vi "New.vi"() -> ()   [LabVIEW 2020, in "MeasurementService Editor.lvlib"]
uses:
  _Editor/MeasurementService Editor.lvlib
panel:
  out "Status":string
  in  "Create Measurement Service":bool
  in  "Measurement Service Name":string
  out "Active Project Name":string
  # "* Project in which Measurement Service will be created"
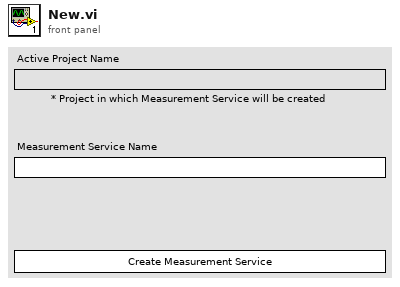
[diagram p1: front panel]
types:
  T1 = enum8{"Enabled", "Disabled", "Disabled and Grayed Out"}
  T2 = cluster{"Project ref":refnum<vi>, "Measurement Service Name":string}
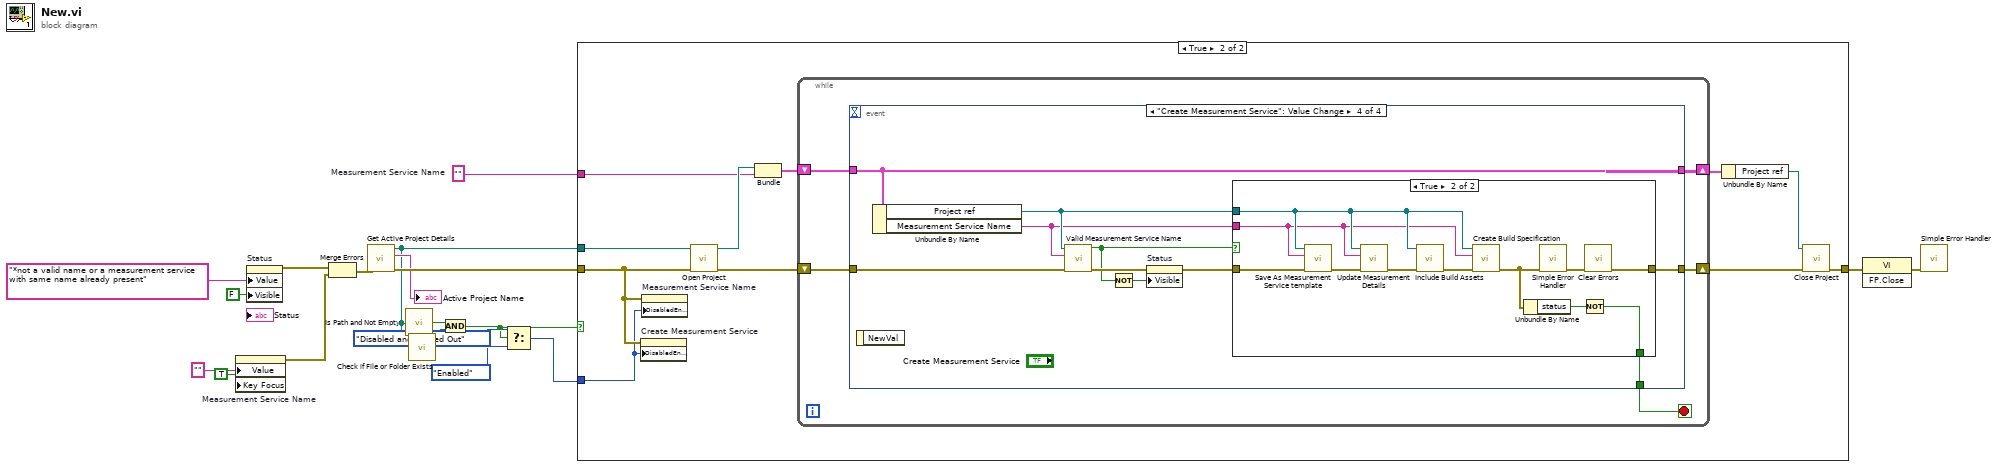
[diagram p0: block diagram]
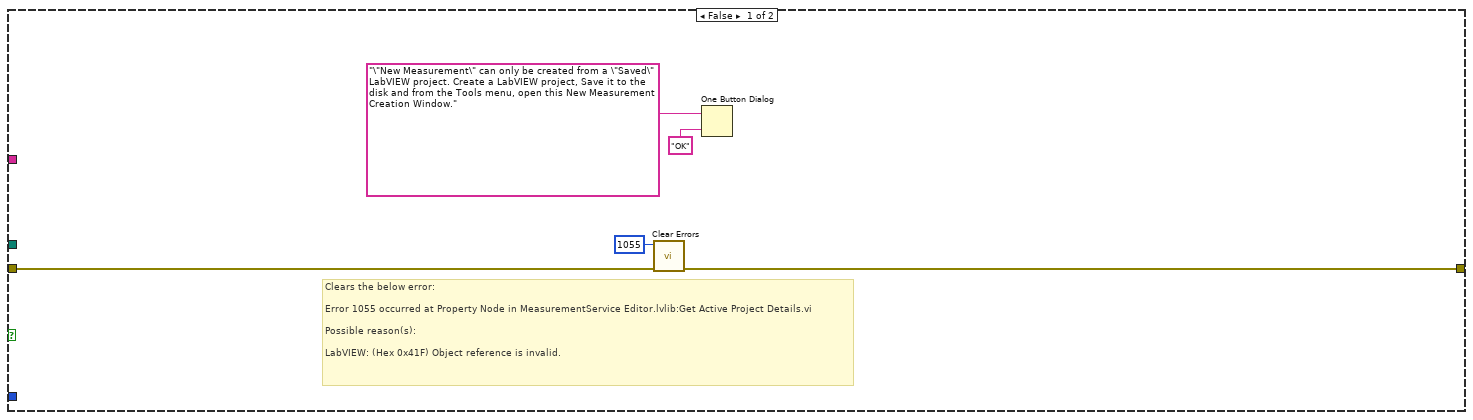
[diagram p2: hidden frame]
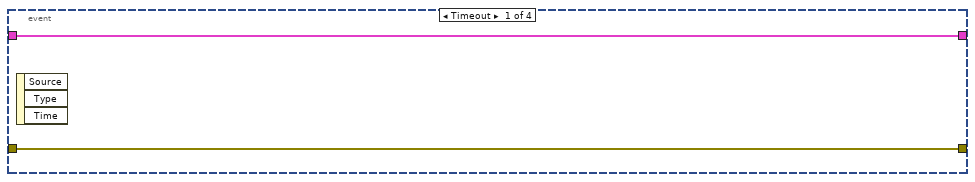
[diagram p3: hidden frame]
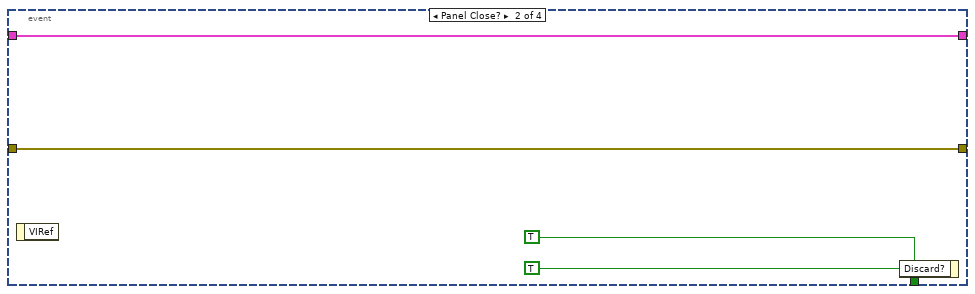
[diagram p4: hidden frame]
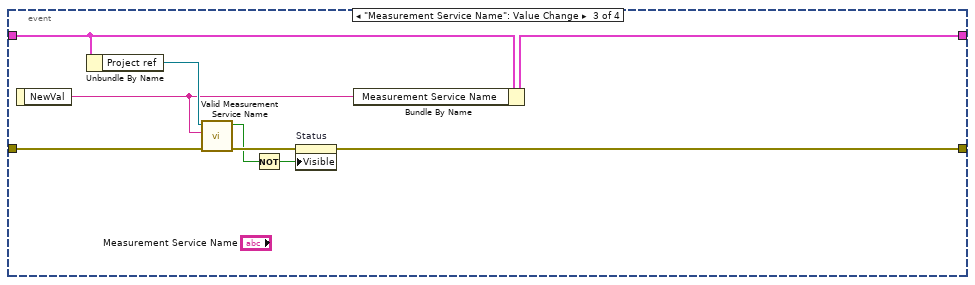
[diagram p5: hidden frame]
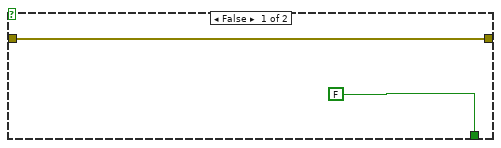
[diagram p6: hidden frame]
diagram:
  w19 = ""  # Measurement Service Name
  n1 = property on="Measurement Service Name" class="Str"("Value"="" ("Measurement Service Name"), "Key Focus"=TRUE) -> (error out=w14:errorcluster)  [unwired: 2 in, 1 out]
  n2 = property on="Status" class="Str"("Value"="*not a valid name or a measurement service with same name already present" ("Status"), "Visible"=FALSE) -> (error out=w16:errorcluster)  [unwired: 2 in, 1 out]
  n3 = Merge Errors(w16, w14) -> (w15:errorcluster)
  n4 = call "Get Active Project Details.vi"("error in"=w15) -> ("error out"=w10:errorcluster, "Name"=→"Active Project Name":string, "Path"=w5:path)  [unwired: 8 in]
  n5 = call <vilib>:"Is Path and Not Empty.vi"("path"=w5) -> ("Is Path and Not Empty?"=w4:bool)  [unwired: 4 in]
  n6 = call <vilib>:"Check if File or Folder Exists.vi"("path"=w5) -> ("file or folder exists?"=w3:bool)  [unwired: 8 in, 2 out]
  n7 = And(x=w4, y=w3) -> (x .and. y?=w2:bool)
  n8 = Select(t=T1."Enabled" ("Disabled"), s=w2, f=T1."Disabled and Grayed Out" ("Disabled")) -> (s? t:f=w6:T1)
  n9 = case shown="True" w2 {
    tunnel: w19 -> [_ w29]
    tunnel: [w21 w28] -> w12
    tunnel: w10 -> [w24 w27]
    tunnel: w6 -> [_ w26]
    tunnel: w5 -> [_ w25]
    frame False {
      # "Clears the below error:\n\nError 1055 occurred at Property Node in MeasurementService Editor.lvlib:Get Active Project Details.vi\n\nPossible reason(s):\n\nLabVIEW: (Hex 0x41F) Object reference is invalid."
      n10 = call <vilib>:"Clear Errors.vi"("error in (no error)"=w24, "specific error code to clear (0: all)"=1055) -> ("error out"=w21:errorcluster)  [unwired: 4 in, 1 out]
      n11 = One Button Dialog(message="\"New Measurement\" can only be created from a \"Saved\" LabVIEW project. Create a LabVIEW project, Save it to the disk and from the Tools menu, open this New Measurement Creation Window.", button name ("OK")="OK") -> ()  [unwired: 1 out]
    }
    frame True {
      n12 = property on="Create Measurement Service" class="Bool"(error in=w27, "DisabledEnum"=w26) -> ()  [unwired: 1 in, 2 out]
      n13 = property on="Measurement Service Name" class="Str"(error in=w27, "DisabledEnum"=w26) -> ()  [unwired: 1 in, 2 out]
      n14 = call "Open Project.vi"("error in"=w27, "Path"=w25) -> ("error out"=w35:errorcluster, "Project ref"=w34:refnum<vi>)  [unwired: 8 in]
      n15 = Bundle("Project ref"=w34, "Measurement Service Name"=w29) -> (w33:T2)  [unwired: 1 in]
      n16 = while {
        shift-right: [w39] -> w30
        shift-left: w35 -> [w38]
        shift-right: [w36] -> w32
        shift-left: w33 -> [w37]
        stop <- w40 stop-if-true
        n17 = event shown="[3] \"Create Measurement Service\": Value Change" {
          selector: _ -> [_ _ _ _]
          dyn-events: _ -> [_ _ _ _]
          timeout: _ -> [_ _ _ _]
          tunnel: [_ TRUE ("Discard?") _ w58] -> w40
          tunnel: [w42 w44 w50 w59] -> w39
          tunnel: w38 -> [w42 w44 w51 w64]
          tunnel: w37 -> [w41 w43 w49 w65]
          tunnel: [w41 w43 w55 w65] -> w36
          event Timeout {
            n18 = event-data() -> ()  [unwired: 1 in, 3 out]
          }
          event Panel Close? {
            n19 = event-data() -> ()  [unwired: 1 in, 1 out]
            n20 = event-data("Discard?"=TRUE) -> ()  [unwired: 1 in, 1 out]
          }
          event "Measurement Service Name": Value Change {
            n21 = event-data() -> ("NewVal"=w47:string)  [unwired: 1 in]
            n22 = Unbundle By Name(w49) -> ("Project ref"=w48:refnum<vi>)
            n23 = call "Valid Measurement Service Name.vi"("error in"=w51, "Valid Service Name"=w47, "Project ref"=w48) -> ("error out"=w54:errorcluster, "Valid Name?"=w52:bool)  [unwired: 7 in]
            n24 = Not(x=w52) -> (.not. x?=w53:bool)
            n25 = property on="Status" class="Str"(error in=w54, "Visible"=w53) -> (error out=w50:errorcluster)  [unwired: 1 in, 1 out]
            n26 = Bundle By Name(cluster=w49, "Measurement Service Name"=w47) -> (w55:T2)
          }
          event "Create Measurement Service": Value Change {
            n27 = event-data() -> ()  [unwired: 1 in, 1 out]
            n28 = Unbundle By Name(w65) -> ("Project ref"=w57:refnum<vi>, "Measurement Service Name"=w56:string)
            n29 = call "Valid Measurement Service Name.vi"("error in"=w64, "Valid Service Name"=w56, "Project ref"=w57) -> ("error out"=w63:errorcluster, "Valid Name?"=w61:bool)  [unwired: 7 in]
            n30 = Not(x=w61) -> (.not. x?=w62:bool)
            n31 = property on="Status" class="Str"(error in=w63, "Visible"=w62) -> (error out=w60:errorcluster)  [unwired: 1 in, 1 out]
            n32 = case shown="True" w61 {
              tunnel: w60 -> [w67 w78]
              tunnel: [w67 w74] -> w59
              tunnel: [FALSE w76] -> w58
              tunnel: w57 -> [_ w69]
              tunnel: w56 -> [_ w68]
              frame False {
              }
              frame True {
                n33 = call "Save As Measurement Service template.vi"("error in"=w78, "Measurement Service Name"=w68, "Project ref"=w69) -> ("error out"=w73:errorcluster)  [unwired: 8 in]
                n34 = call "Update Measurement Details.vi"("error in"=w73, "Measurement Service Name"=w68, "Project ref"=w69) -> ("error out"=w72:errorcluster)  [unwired: 8 in]
                n35 = call "Include Build Assets.vi"("error in"=w72, "Project ref"=w69) -> ("error out"=w71:errorcluster)  [unwired: 9 in]
                n36 = call "Create Build Specification.vi"("error in (no error)"=w71, "Measurement Service Name"=w68, "Project in"=w69) -> ("error out"=w70:errorcluster)  [unwired: 8 in]
                n37 = Unbundle By Name(w70) -> ("status"=w77:bool)
                n38 = call <vilib>:"Simple Error Handler.vi"("error in (no error)"=w70) -> ("error out"=w75:errorcluster)  [unwired: 4 in, 4 out]
                n39 = Not(x=w77) -> (.not. x?=w76:bool)
                n40 = call <vilib>:"Clear Errors.vi"("error in (no error)"=w75) -> ("error out"=w74:errorcluster)  [unwired: 5 in, 1 out]
              }
            }
          }
        }
      }
      n41 = Unbundle By Name(w32) -> ("Project ref"=w31:refnum<vi>)
      n42 = call "Close Project.vi"("error in"=w30, "Project ref"=w31) -> ("error out"=w28:errorcluster)  [unwired: 9 in]
    }
  }
  n43 = invoke class="VI" method="FP.Close"(error in=w12) -> (error out=w11:errorcluster)  [unwired: 2 in, 2 out]
  n44 = call <vilib>:"Simple Error Handler.vi"("error in (no error)"=w11) -> ()  [unwired: 4 in, 5 out]
